vi "Read Size Width.vi"(8 "error in (no error)":errorcluster, 11 "IOName.lvclass in":refnum<class "IOName.lvclass">) -> (0 "error out":errorcluster, 2 "Width":u32, 3 "IOName.lvclass out":refnum<class "IOName.lvclass">)   [LabVIEW 2015, in "IOName.lvclass"]
uses:
  IOName.lvclass
  IOName.lvclass/IOName.ctl
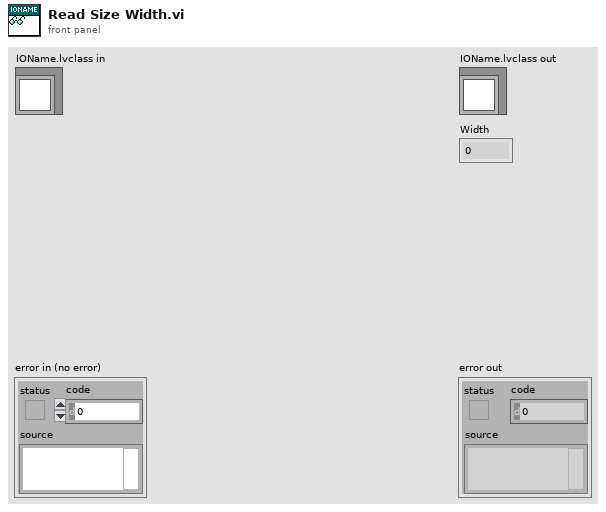
[diagram p1: front panel]
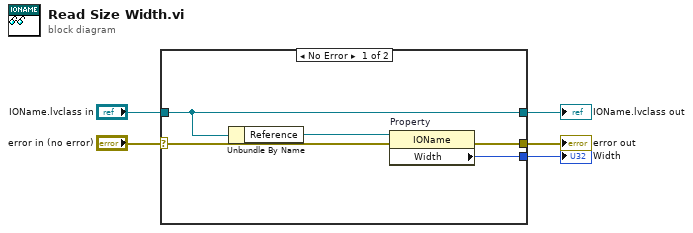
[diagram p0: block diagram]
diagram:
  n1 = case shown="No Error" "error in (no error)" {
    selector: "error in (no error)" -> [w6 w12]
    tunnel: [w9 w12] -> w4
    tunnel: [w8 w11] -> w2
    tunnel: "IOName.lvclass in" -> [w8 w11]
    tunnel: [w10 _] -> w1
    frame No Error {
      n2 = Unbundle By Name(w8) -> ("Reference"=w7:refnum<vi>)
      n3 = property on="Property" class="IOName"(reference=w7, error in=w6) -> (error out=w9:errorcluster, "Width"=w10:u32)  [unwired: 1 out]
    }
    frame Error {
    }
  }
  "error out" <- w4
  "IOName.lvclass out" <- w2
  "Width" <- w1
